vi "PathFollower.vi"(0 "Waypoint 2":dbl[](array[numeric]), 1 "Position":dbl[](array[numeric]), 2 "Dest":dbl[](array[numeric]), 3 "Reinitialize":bool, 5 "Waypoint 1":dbl[](array[numeric]), 9 "Waypoint 0":dbl[](array[numeric]), 11 "Dest_orientation":dbl, 12 "output xy":dbl=1.0, 13 "output angle":dbl=4.0, 15 "dest_vel":dbl) -> (4 "Output\nVelocity":dbl[](array[numeric]) format="%.2f")   [LabVIEW 2017]
uses:
  <vilib>/Analysis/_algsub.llb/Real Vector Norm.vi
  <vilib>/Analysis/coordinate.llb/Wrap Angle (scalar).vi
  <vilib>/Analysis/coordinate.llb/2D Cartesian Coordinate Rotation (Scalar).vi
  <vilib>/Analysis/NI_AALPro.lvlib
  <vilib>/Analysis/NI_AAL_Angle.lvlib
panel:
  out "abs(x)":dbl
  in  "PID gains paralelo":T1={"proportional gain (Kc)"=0.007, "integral time (Ti, min)"=0.0, "derivative time (Td, min)"=-0.07}
  out "output array":cluster{"output high":dbl, "output low":dbl}[](array[cluster])
  in  "PID Gains Angle":T1={"proportional gain (Kc)"=5.0, "integral time (Ti, min)"=0.0, "derivative time (Td, min)"=-2.0}
  in  "PID Gains lateral":T1={"proportional gain (Kc)"=0.01, "integral time (Ti, min)"=0.0, "derivative time (Td, min)"=-0.07}
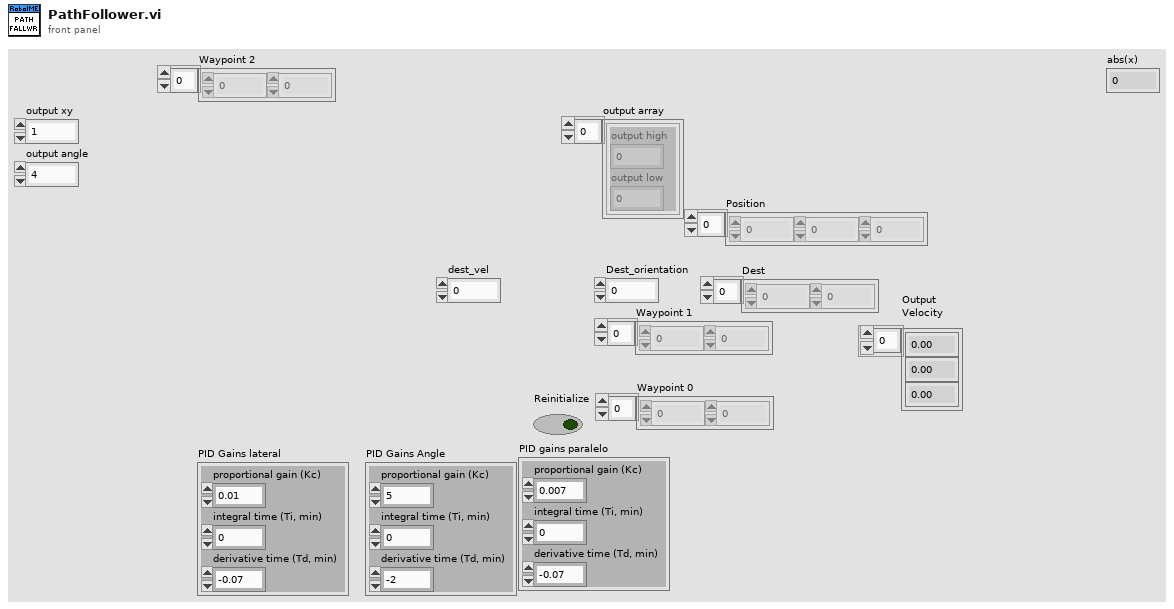
[diagram p1: front panel]
types:
  T1 = cluster{"proportional gain (Kc)":dbl, "integral time (Ti, min)":dbl, "derivative time (Td, min)":dbl}
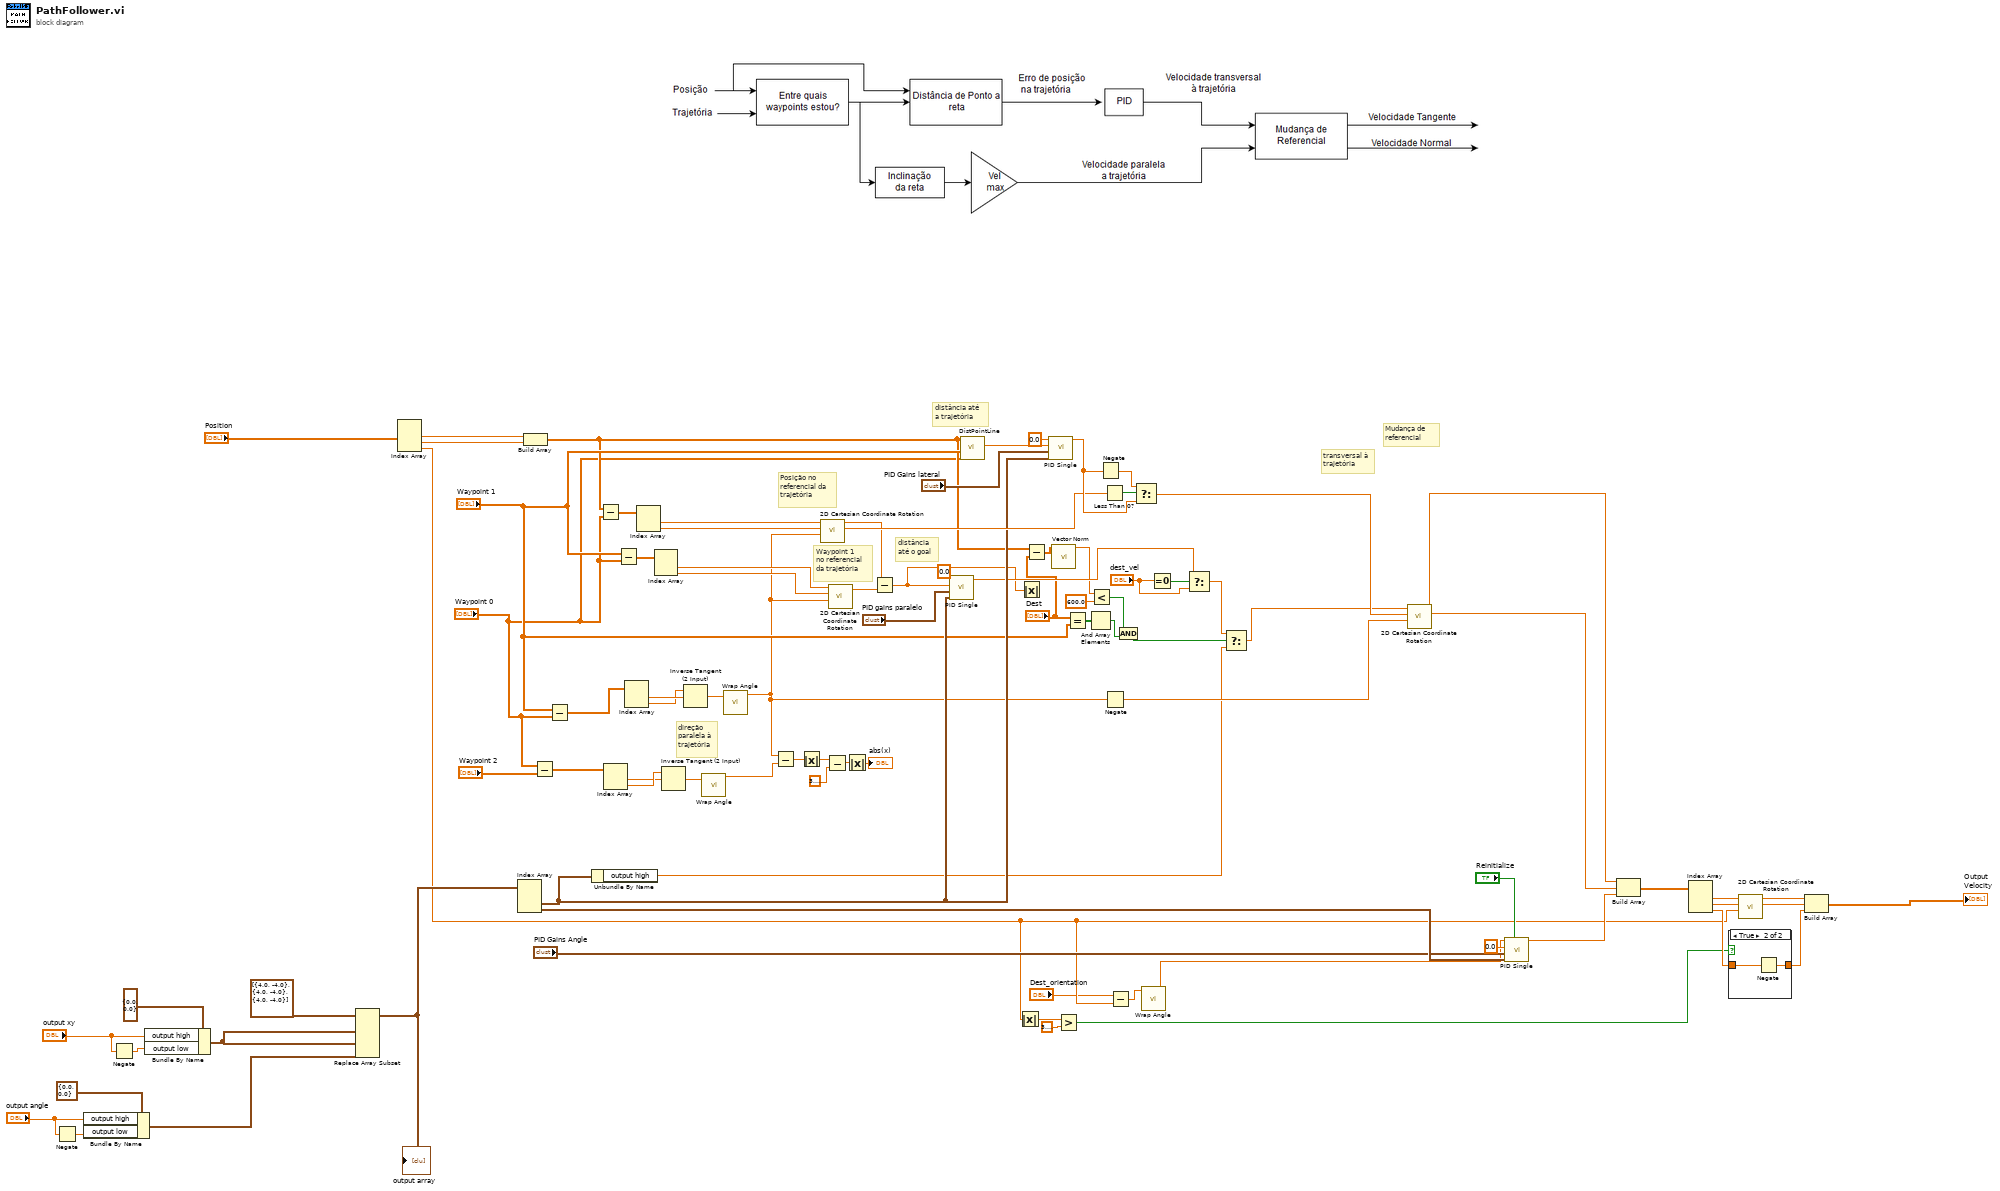
[diagram p0: block diagram]
diagram:
  # "Waypoint 1\nno referencial\nda trajetória"
  # "Posição no \nreferencial da\ntrajetória"
  # "distância \naté o goal"
  # "distância até \na trajetória"
  # "Mudança de \nreferencial"
  # "transversal à\ntrajetória"
  # "direção\nparalela à\ntrajetória"
  n1 = Negate(x="output angle") -> (-x=w65:dbl)
  n2 = Bundle By Name(cluster=cluster{"output high":dbl, "output low":dbl} {"output high"=0.0, "output low"=0.0}, "output high"="output angle", "output low"=w65) -> (w71:cluster{"output high":dbl, "output low":dbl})
  n3 = Negate(x="output xy") -> (-x=w67:dbl)
  n4 = Bundle By Name(cluster=cluster{"output high":dbl, "output low":dbl} {"output high"=0.0, "output low"=0.0} ("new element/subarray"), "output high"="output xy", "output low"=w67) -> (w69:cluster{"output high":dbl, "output low":dbl})
  n5 = Replace Array Subset(array=cluster{"output high":dbl, "output low":dbl}[] [{"output high"=4.0, "output low"=-4.0}, {"output high"=4.0, "output low"=-4.0}, {"output high"=4.0, "output low"=-4.0}] ("output range"), new element #1=w69, new element #2=w69, new element #3=w71) -> (w68:cluster{"output high":dbl, "output low":dbl}[])  [unwired: 3 in]
  "output array" <- w68
  n6 = Index Array(array="Position") -> (element #1=w53:dbl, element #2=w52:dbl, element #3=w62:dbl)  [unwired: 3 in]
  n7 = Index Array(array=w68) -> (element #2=w31:cluster{"output high":dbl, "output low":dbl}, element #3=w79:cluster{"output high":dbl, "output low":dbl})  [unwired: 3 in, 1 out]
  n8 = Build Array(w53, w52) -> (w16:dbl[])
  n9 = Subtract(x="Waypoint 0", y="Waypoint 2") -> (x-y=w8:dbl[])
  n10 = Subtract(x="Waypoint 1", y="Waypoint 0") -> (x-y=w40:dbl[])
  n11 = Unbundle By Name(w31) -> ("output high"=w28:dbl)
  n12 = Subtract(x=w16, y="Waypoint 0") -> (x-y=w47:dbl[])
  n13 = Index Array(array=w8) -> (element #1=w9:dbl, element #2=w11:dbl)  [unwired: 2 in]
  n14 = Subtract(x="Waypoint 1", y="Waypoint 0") -> (x-y=w38:dbl[])
  n15 = Index Array(array=w40) -> (element #1=w55:dbl, element #2=w39:dbl)  [unwired: 2 in]
  n16 = Index Array(array=w47) -> (element #1=w46:dbl, element #2=w45:dbl)  [unwired: 2 in]
  n17 = Index Array(array=w38) -> (element #1=w37:dbl, element #2=w36:dbl)  [unwired: 2 in]
  n18 = Inverse Tangent (2 Input)(1:w9, 2:w11) -> (0:w10:dbl)
  n19 = Inverse Tangent (2 Input)(1:w55, 2:w39) -> (0:w54:dbl)
  n20 = call-poly <vilib>:"Wrap Angle.vi"("angle in"=w10) -> ("angle out"=w6:dbl)  [unwired: 9 in, 1 out]
  n21 = call-poly <vilib>:"Wrap Angle.vi"("angle in"=w54) -> ("angle out"=w7:dbl)  [unwired: 9 in, 1 out]
  n22 = Subtract(x=w7, y=w6) -> (x-y=w5:dbl)
  n23 = Absolute Value(x=w5) -> (abs(x)=w4:dbl)
  n24 = call-poly <vilib>:"2D Cartesian Coordinate Rotation.vi"("theta"=w7, "y"=w45, "x"=w46) -> ("y out"=w48:dbl, "x out"=w35:dbl)  [unwired: 6 in, 1 out]
  n25 = Subtract(x=w4, y=3.141592653589793) -> (x-y=w1:dbl)
  n26 = call-poly <vilib>:"2D Cartesian Coordinate Rotation.vi"("theta"=w7, "y"=w36, "x"=w37) -> ("x out"=w34:dbl)  [unwired: 6 in, 2 out]
  n27 = Absolute Value(x=w1) -> (abs(x)=→"abs(x)":dbl)
  n28 = Subtract(x=w35, y=w34) -> (x-y=w19:dbl)
  n29 = call "PID Single.vi"("Limits"=w31, "PID gains in"="PID gains paralelo", "Variable"=w19, "Setpoint"=0.0) -> ("Out"=w22:dbl)  [unwired: 7 in]
  n30 = call "DistPointLine.vi"("P2"="Waypoint 0", "P1"="Waypoint 1", "Q"=w16) -> ("distance"=w61:dbl)  [unwired: 8 in]
  n31 = Absolute Value(x=w62) -> (abs(x)=w85:dbl)
  n32 = Absolute Value(x=w19) -> ()  [unwired: 1 out]
  n33 = Subtract(x=w16, y="Dest") -> (x-y=w18:dbl[])
  n34 = call "PID Single.vi"("Limits"=w31, "PID gains in"="PID Gains lateral", "Variable"=w61, "Setpoint"=0.0) -> ("Out"=w50:dbl)  [unwired: 7 in]
  n35 = call-poly <vilib>:"Vector Norm.vi"("Input Vector"=w18) -> ("norm"=w15:dbl)  [unwired: 9 in, 1 out]
  n36 = Greater?(x=w85, y=3.141592653589793) -> (0:w80:bool)
  n37 = Equal?(x="Dest", y="Waypoint 1") -> (x = y?=w29:bool[])
  n38 = And Array Elements(Boolean array=w29) -> (logical AND=w14:bool)
  n39 = Less?(x=w15, y=600.0) -> (x < y?=w24:bool)
  n40 = Negate(x=w50) -> (-x=w51:dbl)
  n41 = Less Than 0?(x=w48) -> (x < 0?=w44:bool)
  n42 = Negate(x=w7) -> (-x=w58:dbl)
  n43 = Subtract(x="Dest_orientation", y=w62) -> (x-y=w76:dbl)
  n44 = Compound Arithmetic op=AND(w24, w14) -> (w26:bool)
  n45 = Select(t=w51, s=w44, f=w50) -> (s? t:f=w49:dbl)
  n46 = call-poly <vilib>:"Wrap Angle.vi"("angle in"=w76) -> ("angle out"=w75:dbl)  [unwired: 9 in, 1 out]
  n47 = Equal To 0?(x="dest_vel") -> (x = 0?=w23:bool)
  n48 = Select(t=w22, s=w23, f="dest_vel") -> (s? t:f=w20:dbl)
  n49 = Select(t=w20, s=w26, f=w28) -> (s? t:f=w27:dbl)
  n50 = call-poly <vilib>:"2D Cartesian Coordinate Rotation.vi"("theta"=w58, "y"=w49, "x"=w27) -> ("y out"=w56:dbl, "x out"=w57:dbl)  [unwired: 6 in, 1 out]
  n51 = call "PID Single.vi"("initialize"="Reinitialize", "Limits"=w79, "PID gains in"="PID Gains Angle", "Variable"=0.0, "Setpoint"=w75) -> ("Out"=w81:dbl)  [unwired: 6 in]
  n52 = Build Array(w57, w56, w81) -> (w74:dbl[])
  n53 = Index Array(array=w74) -> (element #1=w89:dbl, element #2=w88:dbl, element #3=w84:dbl)  [unwired: 3 in]
  n54 = case shown="True" w80 {
    tunnel: w84 -> [w90 w92]
    tunnel: [w90 w91] -> w83
    frame False {
    }
    frame True {
      n55 = Negate(x=w92) -> (-x=w91:dbl)
    }
  }
  n56 = call-poly <vilib>:"2D Cartesian Coordinate Rotation.vi"("theta"=w62, "y"=w88, "x"=w89) -> ("y out"=w86:dbl, "x out"=w87:dbl)  [unwired: 6 in, 1 out]
  n57 = Build Array(w87, w86, w83) -> (→"Output\nVelocity":dbl[])
